vi "Convert Z norm factor to fractional binary.vi"() -> (3 "Fractional Z norm factor":u8 format="%08b")   [LabVIEW 2020]
uses:
  Global Variables/General Globals.vi
panel:
  out "x/y":dbl
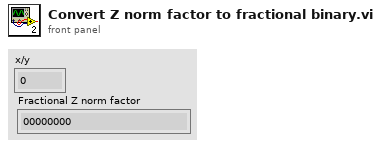
[diagram p1: front panel]
types:
  T1 = enum16{"Initialise", "Load from file", "Save to file", "Read", "Write"}
  T2 = typedef "Calibration config.ctl" = cluster{"Current Objective":string, "Objective Settings":T3[], "PreChirper Values Preset ?":bool, "PreChirper Settings":T4[], "PreChirper Constants":T5}
  T3 = typedef "Objective Config.ctl" = cluster{"Name":string, "Sum X":dbl, "Sum Y":dbl, "Diff X":dbl, "Diff Y":dbl, "Distortion Correction":dbl, "Z_norm to um_scaling":dbl, "X_norm to um_scaling":dbl, "Calibrated Wavelength":dbl}
  T4 = typedef "Prechirper Cal Config.ctl" = cluster{"Wavelength":i32, "Prism 1":i32, "Prism 2":i32}
  T5 = typedef "PreChirper constants.ctl" = cluster{"a 1":i32, "b 1":i32, "c 1":i32, "a 2":i32, "b 2":i32, "c 2":i32, "lmin":i32, "lmax":i32}
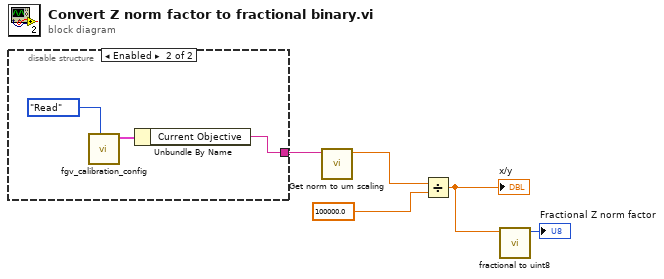
[diagram p0: block diagram]
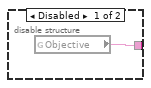
[diagram p2: hidden frame]
diagram:
  n1 = disable-structure shown="Enabled" {
    disable-tunnel: [w6 w7] -> w4
    frame Disabled {
      n2 = global read "General Globals.vi" "Objective"() -> (w6:string)
    }
    frame Enabled {
      n3 = call "fgv_calibration_config.vi"("Cal config ops"=T1."Read") -> ("Config cluster OUT"=w9:T2)  [unwired: 8 in, 2 out]
      n4 = Unbundle By Name(w9) -> ("Current Objective"=w7:string)
    }
  }
  n5 = call "Get norm to um scaling .vi"("Current Objective"=w4) -> ("Z_norm to um_scaling"=w3:dbl)  [unwired: 7 in, 3 out]
  n6 = Divide(x=w3, y=100000.0) -> (x/y=w2:dbl)
  "x/y" <- w2
  n7 = call "fractional to uint8.vi"("x"=w2) -> ("U8 number"=→"Fractional Z norm factor":u8)  [unwired: 10 in]
